vi "Histogram GUID Lookup.vi"() -> ()   [LabVIEW 2012, in "Histogram Custom Device.lvlib"]
doc: "Use this Global VI to access the GUIDs assigned to the page resources of the Custom Device."
uses:
  Histogram Custom Device.lvlib
panel:
  in  "Custom Device":string="01c4c187-fa58-4953-904c-70165a523d39"
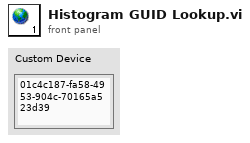
[diagram p1: front panel]
diagram:
